vi "Test Configure.vi"(0 "Template Tx Test in":refnum<class "niDTS BT Tx Test.lvclass">, 11 "error in (no error)":errorcluster) -> (4 "Template Tx Test out":refnum<class "niDTS BT Tx Test.lvclass">, 15 "error out":errorcluster)   [LabVIEW 2015, in "niDTS BT.lvlib" / "niDTS BT Tx Test.lvclass"]
uses:
  niDTS BT Tx Test.lvclass
  Dut/Includes/niDTS BT Dut INC Handle.ctl
  Dut/Objects/BASE_class/niDTS BT Dut.lvclass
  niDTS BT Tx Test.lvclass/niDTS BT Tx Test.ctl
  RiviInstDriver/InstDriver/Objects/InstDriver.lvclass/InstDriver.ctl
  RiviInstDriver/InstDriver/Objects/Read VISA resource.vi
  RiviInstDriver/InstDriver/Objects/Set VISA Read (Byte Count).vi
  TestStand/Station/Objects/SystemTechnologyCatalog/niDTS SystemTechnologyCatalog.lvclass
  TestStand/Station/Objects/SystemDut/niDTS SystemDut.lvclass
  Framework/Dut/Objects/BASE_class/niDTS Dut.lvclass
  Instrument/INSTR TX/niDTS BT INSTR TX.lvclass
  Framework/niDTS Framework.lvlib
  niDTS BT.lvlib
  TestStand/niDTS TestStand.lvlib
  RiviInstDriver/InstDriver/Objects/InstDriver.lvclass
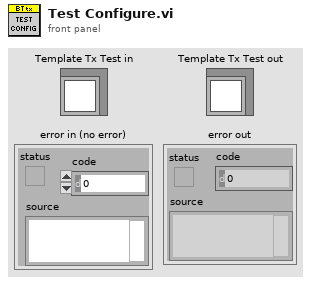
[diagram p1: front panel]
types:
  T1 = typedef "niDTS BT.lvlib/niDTS BT Dut INC Handle.ctl" = refnum<data-value>
  T2 = typedef "niDTS Framework.lvlib/niDTS Dut INC Handle.ctl" = refnum<data-value>
  T3 = typedef "niDTS BT.lvlib/niDTS BT Tx Test INC Parameters.ctl" = cluster{"Channel":i32, "Data Rate ":i32, "Dut Tx Power":dbl, "External Attenuation (dB)":dbl[], "Auto Level":bool, "Packet type":T4, "Payload Pattern":T5, "Burst Sync":enum16{"NONE", "PREamble"}, "BD ADDRESS":u32, "Packet Length, bytes":i32, "ModAcc Measurement Paramaters":cluster{"ModAcc Enable":bool, "CFO Enable":bool, "Character Select":T6, "Averages":i32, "Averaging Mode":enum16{"RMS", "LOG", "SCALAR", "MAX", "MIN", "VECTOR"}, "Measurement Length":i32, "Measurement Offset":i32}, "OBW Measurement Parameters":T7, "TXP Measurement Parameters":T8, "IBE  Measurement Parameters":T9, "Trace Enable":bool, "Trigger":T10}
  T4 = typedef "niDTS BT.lvlib/niDTS BT INC Packet Type.ctl" = enum16{"NULL", "POLL", "FHS", "DM1", "DH1", "HV1", "HV2", "HV3", "EV3", "DV", "AUX1", "DM3", "DH3", "EV4", "EV5", "DM5", "DH5", "LE-TP"}
  T5 = typedef "niDTS BT.lvlib/niDTS BT Tx Test INC BD Payload Data.ctl" = enum16{"0", "1", "01", "00001111", "PN9", "AUTO"}
  T6 = typedef "niDTS BT.lvlib/niDTS BT Tx Test INC Modulation Characteristics.ctl" = enum16{"DF1", "DF2", "BOTH"}
  T7 = typedef "niDTS BT.lvlib/niDTS BT INC OBW Measurement Parameters.ctl" = cluster{"OBW Enable":bool, "OBW Averages":i32, "Averaging Type":enum16{"RMS", "LOG", "SCALAR", "MAX", "MIN", "VECTOR"}, "Measurement Interval Mode":enum16{"AUTO", "MANUAL"}, "Measurement Interval Length (sec)":dbl}
  T8 = typedef "niDTS BT.lvlib/niDTS BT INC TXP Measurement Parameters.ctl" = cluster{"TXP Power Enable":bool, "TXP Averages":i32, "Averaging Type":enum16{"RMS", "LOG", "SCALAR", "MAX", "MIN"}}
  T9 = typedef "niDTS BT.lvlib/niDTS BT INC EDR IBE Measurement Parameters.ctl" = cluster{"IBE Enable":bool, "IBE Averages":i32, "Averaging Type":enum16{"RMS", "LOG", "SCALAR", "MAX", "MIN", "VECTOR"}, "Numbe of Channels":i32, "Channel Mode":enum16{"InBand", "Centered"}, "Measurement Interval Mode":enum16{"AUTO", "MANUAL"}, "Measurement Interval Length (sec)":dbl}
  T10 = typedef "niDTS BT.lvlib/niDTS BT DUT INC Trigger.ctl" = cluster{"MinQuietTimeDuration (sec)":dbl, "TriggerDelay (sec)":dbl, "TriggerEdge":enum16{"RISing", "FALLing"}, "TriggerSource":enum16{"IMMediate", "RF0", "PFI0", "PFI1", "RTS0", "RTS1", "RTS2", "RTS3", "RTS4", "RTS5", "RTS6", "RTS7", "PXIStar", "SOFT"}, "TriggerThreshold (dB)":dbl, "TriggerTimeout (sec)":dbl}
  T11 = typedef "niDTS BT.lvlib/niDTS BT DUT INC Parameters.ctl" = cluster{"Channel":i32, "Pattern":enum16{"0", "1", "01", "00001111", "PN9"}, "Packet type":enum16{"NULL", "POLL", "FHS", "DM1", "DH1", "HV1", "HV2", "HV3", "EV3", "DV", "AUX1", "DM3", "DH3", "EV4", "EV5", "DM5", "DH5", "LE-TP"}, "Power":dbl, "Report Period (ms)":dbl, "BD Address":i64, "Data Rate":enum16{"1", "2", "3"}, "Number of Packets":i32, "Packet Length, bytes":i32}
  T12 = typedef "InstDriver.lvclass/niInstDriver INC Handle.ctl" = refnum<data-value>
  T13 = typedef "niRfsaBt.lvclass/niRfsaBT INC Handle.ctl" = refnum<data-value>
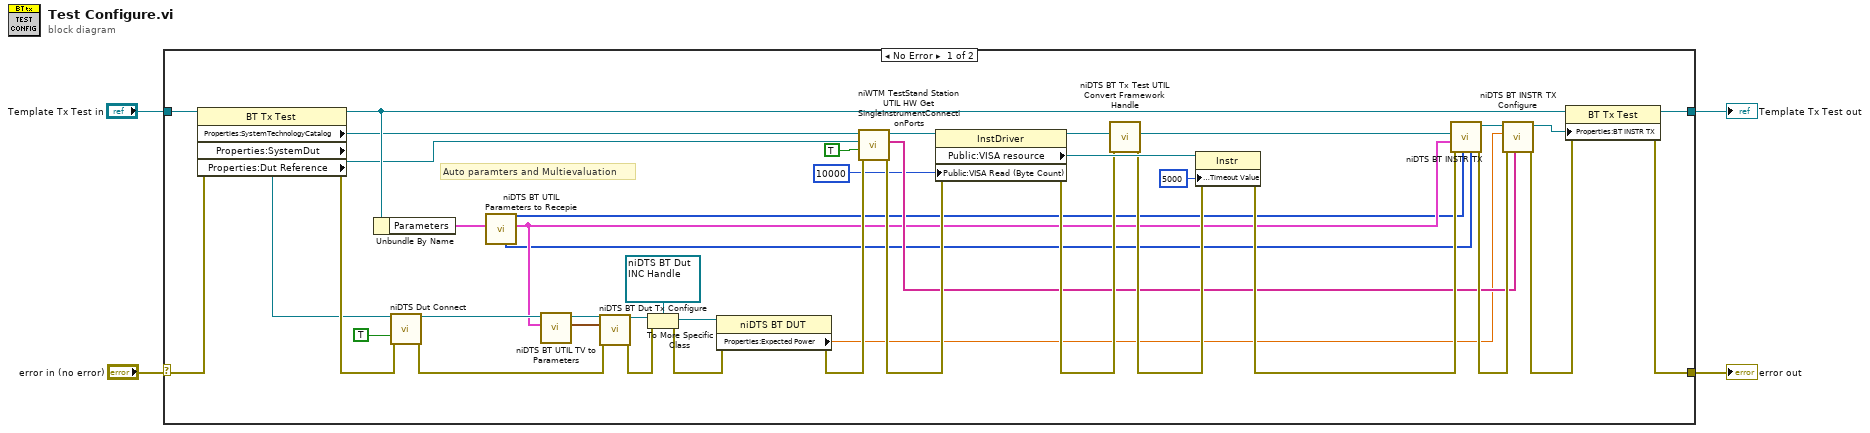
[diagram p0: block diagram]
diagram:
  n1 = case shown="No Error" "error in (no error)" {
    selector: "error in (no error)" -> [w41 w46]
    tunnel: [w31 w46] -> w2
    tunnel: [w33 w45] -> w3
    tunnel: "Template Tx Test in" -> [w44 w45]
    frame No Error {
      # "Auto paramters and Multievaluation"
      n2 = property class="BT Tx Test"(reference=w44, error in=w41) -> (reference out=w29:refnum<class "niDTS BT Tx Test.lvclass">, error out=w39:errorcluster, "Properties:SystemTechnologyCatalog"=w26:refnum<class "niDTS SystemTechnologyCatalog.lvclass">, "Properties:SystemDut"=w27:refnum<class "niDTS SystemDut.lvclass">, "Properties:Dut Reference"=w28:T2)
      n3 = Unbundle By Name(w29) -> ("Parameters"=w8:T3)
      n4 = call "niDTS Dut Connect.vi"("Dut Handle"=w28, "Auto Interface"=TRUE, "error in (no error)"=w39) -> ("Dut Handle out"=w42:T2, "error out"=w40:errorcluster)  [unwired: 11 in]
      n5 = call "niDTS BT UTIL Parameters to Recepie.vi"("BT Tx Parameters"=w8) -> ("BT Tx Parameters Out"=w7:T3, "Payloads"=w5:T5[], "Measurements"=w6:enum16{"Other", "DF1", "DF2"}[])  [unwired: 8 in]
      n6 = call "niDTS BT UTIL TV to Parameters.vi"("BT Tx Parameters"=w7) -> ("niDTS BT DUT Parameters"=w30:T11)  [unwired: 10 in]
      n7 = call "niDTS BT Dut Tx Configure.vi"("Dut Handle in"=w42, "niDTS BT DUT Parameters"=w30, "error in (no error)"=w40) -> ("Dut Handle"=w17:T2, "error out"=w16:errorcluster)  [unwired: 11 in]
      n8 = To More Specific Class(target class=T1 refnum ("BT Dut Handle"), reference=w17, error in=w16) -> (specific class reference=w15:T1, error out=w14:errorcluster)
      n9 = property class="niDTS BT DUT"(reference=w15, error in=w14) -> (error out=w13:errorcluster, "Properties:Expected Power"=w9:dbl)  [unwired: 1 out]
      n10 = call "niWTM TestStand Station UTIL HW Get SingleInstrumentConnectionPorts.vi"("error in (no error)"=w13, "TX Instrument"=TRUE, "SystemDut"=w27, "SystemTechnologyCatalog"=w26) -> ("error out"=w24:errorcluster, "Ports"=w12:string[], "InstDriver Handle"=w23:T12)  [unwired: 5 in]
      n11 = property class="InstDriver"(reference=w23, error in=w24, "Public:VISA Read (Byte Count)"=u32 10000 ("VISA Read (Byte Count)")) -> (reference out=w22:T12, error out=w21:errorcluster, "Public:VISA resource"=w37:refnum<visa-resource-name>)
      n12 = call "niDTS BT Tx Test UTIL Convert Framework Handle.vi"("error in"=w21, "InstDriver Handle"=w22) -> ("error out"=w20:errorcluster, "niRfsaBT"=w10:T13)  [unwired: 8 in]
      n13 = property class="Instr"(reference=w37, error in=w20, "General Settings:Timeout Value"=u32 5000) -> (error out=w36:errorcluster)  [unwired: 1 out]
      n14 = call "niDTS BT INSTR TX.vi"("Payloads"=w5, "Measurements"=w6, "error in (no error)"=w36, "BT Tx Input Parameters"=w7, "reference out"=w10) -> ("error out"=w34:errorcluster, "niDTS BT INSTR TX out"=w35:refnum<class "niDTS BT INSTR TX.lvclass">)  [unwired: 5 in]
      n15 = call-dynamic "niDTS BT INSTR TX Configure.vi"("Ports"=w12, "error in (no error)"=w34, "Expected Power From DUT"=w9, "niDTS BT INSTR TX in"=w35) -> ("error out"=w32:errorcluster, "niDTS BT INSTR TX out"=w19:refnum<class "niDTS BT INSTR TX.lvclass">)  [unwired: 6 in]
      n16 = property class="BT Tx Test"(reference=w29, error in=w32, "Properties:BT INSTR TX"=w19) -> (reference out=w33:refnum<class "niDTS BT Tx Test.lvclass">, error out=w31:errorcluster)
    }
    frame Error {
    }
  }
  "error out" <- w2
  "Template Tx Test out" <- w3
